vi "ui_ClientSrv Query Observer Password.vi"() -> (4 "OKed?":bool, 6 "observer digest":string, 8 "remember out":bool)   [LabVIEW 2012]
doc: "This dialog allows entry of the server's observer password. A valid observer password is required for the client to be able to connect to the server."
uses:
  typedefs/t_ClientSrv Query Observer Password States.ctl
panel:
  in  "remember?":bool
  in  "observer password":string
  in  "cancel":bool
  in  "OK":bool
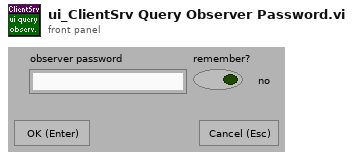
[diagram p1: front panel]
types:
  T1 = typedef "t_ClientSrv Query Observer Password States.ctl" = enum16{"empty queue", "initialize", "stop"}
  T2 = typedef "eventvkey.ctl" = enum16{"ASCII", "Enter", "Return", "Shift", "Ctrl", "Alt", "Cmd", "Opt", "Caps", "NumLock", "Clear", "Break", "Up", "Down", "Left", "Right", "Insert", "Delete", "Home", "End", "PageUp", "PageDown", "Escape", "Help", "Pause", "ScrollLock", "F1", "F2", "F3", "F4", "F5", "F6", "F7", "F8", "F9", "F10", "F11", "F12", "F13", "F14", "F15", "F16", "F17", "F18", "F19", "F20", "F21", "F22", "F23", "F24", "Play", "VolumeUp", "VolumeDown", "Mute", "Two Byte Char"}
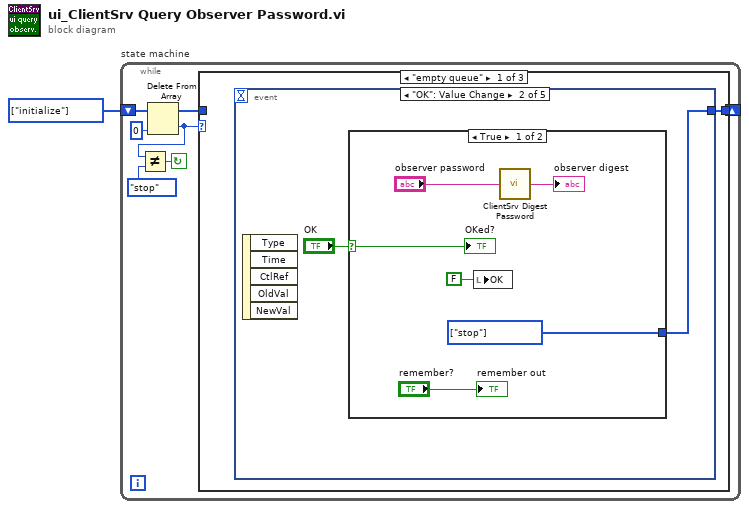
[diagram p0: block diagram]
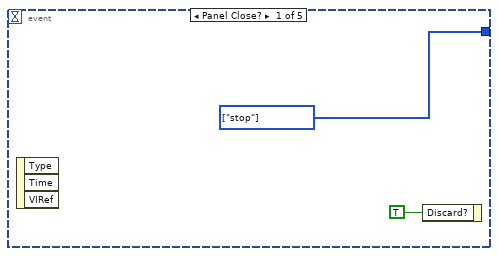
[diagram p2: hidden frame]
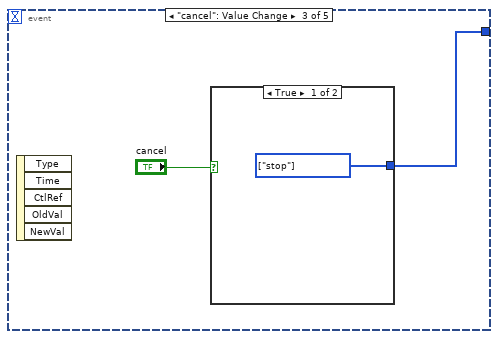
[diagram p4: hidden frame]
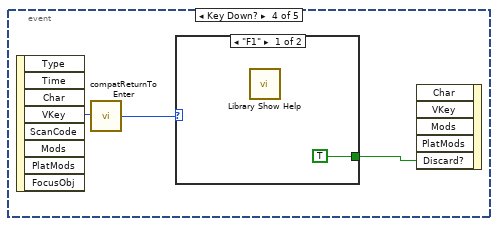
[diagram p6: hidden frame]
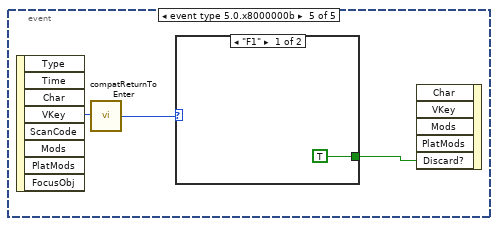
[diagram p8: hidden frame]
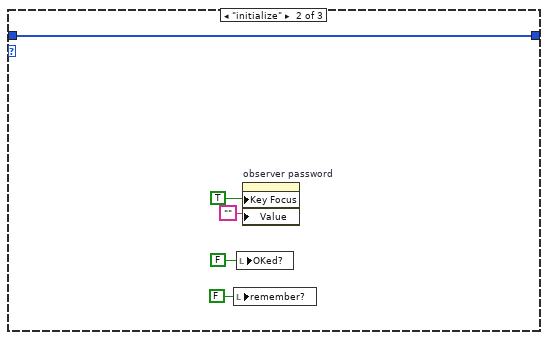
[diagram p10: hidden frame]
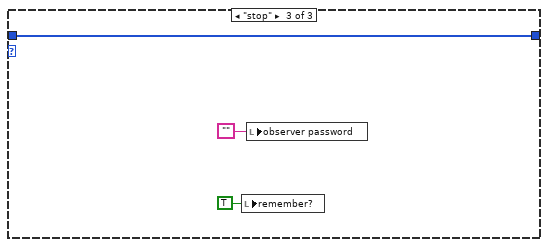
[diagram p11: hidden frame]
diagram:
  w1 = T1[] [enum."initialize"] items=["empty queue", "initialize", "stop"] ("Array Constant")
  n1 = while "state machine" {
    shift-left: w1 -> [w5]
    shift-right: [w8] -> _
    stop <- w7 continue-if-true
    n2 = Delete From Array(array=w5, index=0) -> (deleted portion=w3:T1, array with subset deleted=w4:T1[])  [unwired: 1 in]
    n3 = Not Equal?(x=w3, y=t_ClientSrv_Query_Observer_Password_States."stop" ("states")) -> (x != y?=w7:bool)
    n4 = case "Case" shown="\"empty queue\"" w3 {
      tunnel: [w9 w35 w38] -> w8
      tunnel: w4 -> [_ w35 w38]
      frame "empty queue" {
        n5 = event shown="[1] \"OK\": Value Change" {
          selector: _ -> [_ _ _ _ _]
          dyn-events: _ -> [_ _ _ _ _]
          timeout: _ -> [_ _ _ _ _]
          tunnel: [w11 w13 w21 _ _] -> w9
          event Panel Close? {
            w11 = T1[] [enum."stop"] items=["empty queue", "initialize", "stop"] ("Array Constant")
            n6 = event-data() -> ()  [unwired: 1 in, 3 out]
            n7 = event-data("Discard?"=TRUE) -> ()  [unwired: 1 in, 1 out]
          }
          event "OK": Value Change {
            n8 = event-data() -> ()  [unwired: 1 in, 5 out]
            n9 = case shown="True" "OK" {
              selector: "OK" -> [w18 _]
              tunnel: [w19 _] -> w13
              frame True {
                w19 = T1[] [enum."stop"] items=["empty queue", "initialize", "stop"] ("Array Constant")
                n10 = local write "OK"(FALSE ("OK")) -> ()
                n11 = call "ClientSrv Digest Password.vi"("password"="observer password") -> ("SHA-1 digest"=→"observer digest":string)  [unwired: 14 in]
                "OKed?" <- w18
                "remember out" <- "remember?"
              }
              frame False {
              }
            }
          }
          event "cancel": Value Change {
            n12 = event-data() -> ()  [unwired: 1 in, 5 out]
            n13 = case shown="True" "cancel" {
              tunnel: [w22 _] -> w21
              frame True {
                w22 = T1[] [enum."stop"] items=["empty queue", "initialize", "stop"] ("Array Constant")
              }
              frame False {
              }
            }
          }
          event Key Down? {
            n14 = event-data() -> ("VKey"=w23:T2)  [unwired: 1 in, 7 out]
            n15 = call <vilib>:"compatReturnToEnter.vi"("VKey"=w23) -> ("VKey"=w25:T2)
            n16 = case shown="\"F1\"" w25 {
              tunnel: [TRUE ("Discard?") _] -> w24
              frame "F1" {
                n17 = call "Library Show Help.vi"() -> ()  [unwired: 1 in]
              }
              frame Default {
              }
            }
            n18 = event-data("Discard?"=w24) -> ()  [unwired: 5 in, 1 out]
          }
          event event type 5.0.x8000000b {
            n19 = event-data() -> ("VKey"=w27:T2)  [unwired: 1 in, 7 out]
            n20 = call <vilib>:"compatReturnToEnter.vi"("VKey"=w27) -> ("VKey"=w29:T2)
            n21 = case shown="\"F1\"" w29 {
              tunnel: [TRUE ("Discard?") _] -> w28
              frame "F1" {
              }
              frame Default {
              }
            }
            n22 = event-data("Discard?"=w28) -> ()  [unwired: 5 in, 1 out]
          }
        }
      }
      frame "initialize" {
        n23 = local write "remember?"(FALSE ("remember?")) -> ()
        n24 = local write "OKed?"(FALSE ("OKed?")) -> ()
        n25 = property on="observer password" class="Str"("Key Focus"=TRUE, "Value"="" ("machine name")) -> ()  [unwired: 2 in, 2 out]
      }
      frame "stop" {
        n26 = local write "remember?"(TRUE ("remember?")) -> ()
        n27 = local write "observer password"("") -> ()
      }
    }
  }
